vi "Point Tool Histogram Filter.vi"(4 "Range":cluster{"Lower value":sgl, "Upper value":sgl}={"Lower value"=162.0, "Upper value"=255.0}, 6 "Color threshold limits":T2, 8 "error in":errorcluster, 9 "Combo Box":string(combo), 10 "Subtraction Image":path, 11 "Image in":T1) -> (0 "error out":errorcluster, 3 "Image out":T1)   [LabVIEW 2020]
uses:
  <vilib>/vision/Image Controls.llb/IMAQ Image.ctl
  <vilib>/vision/NI_Vision_Development_Module.lvlib
panel:
  out "Image 2":T1(plugin-control)
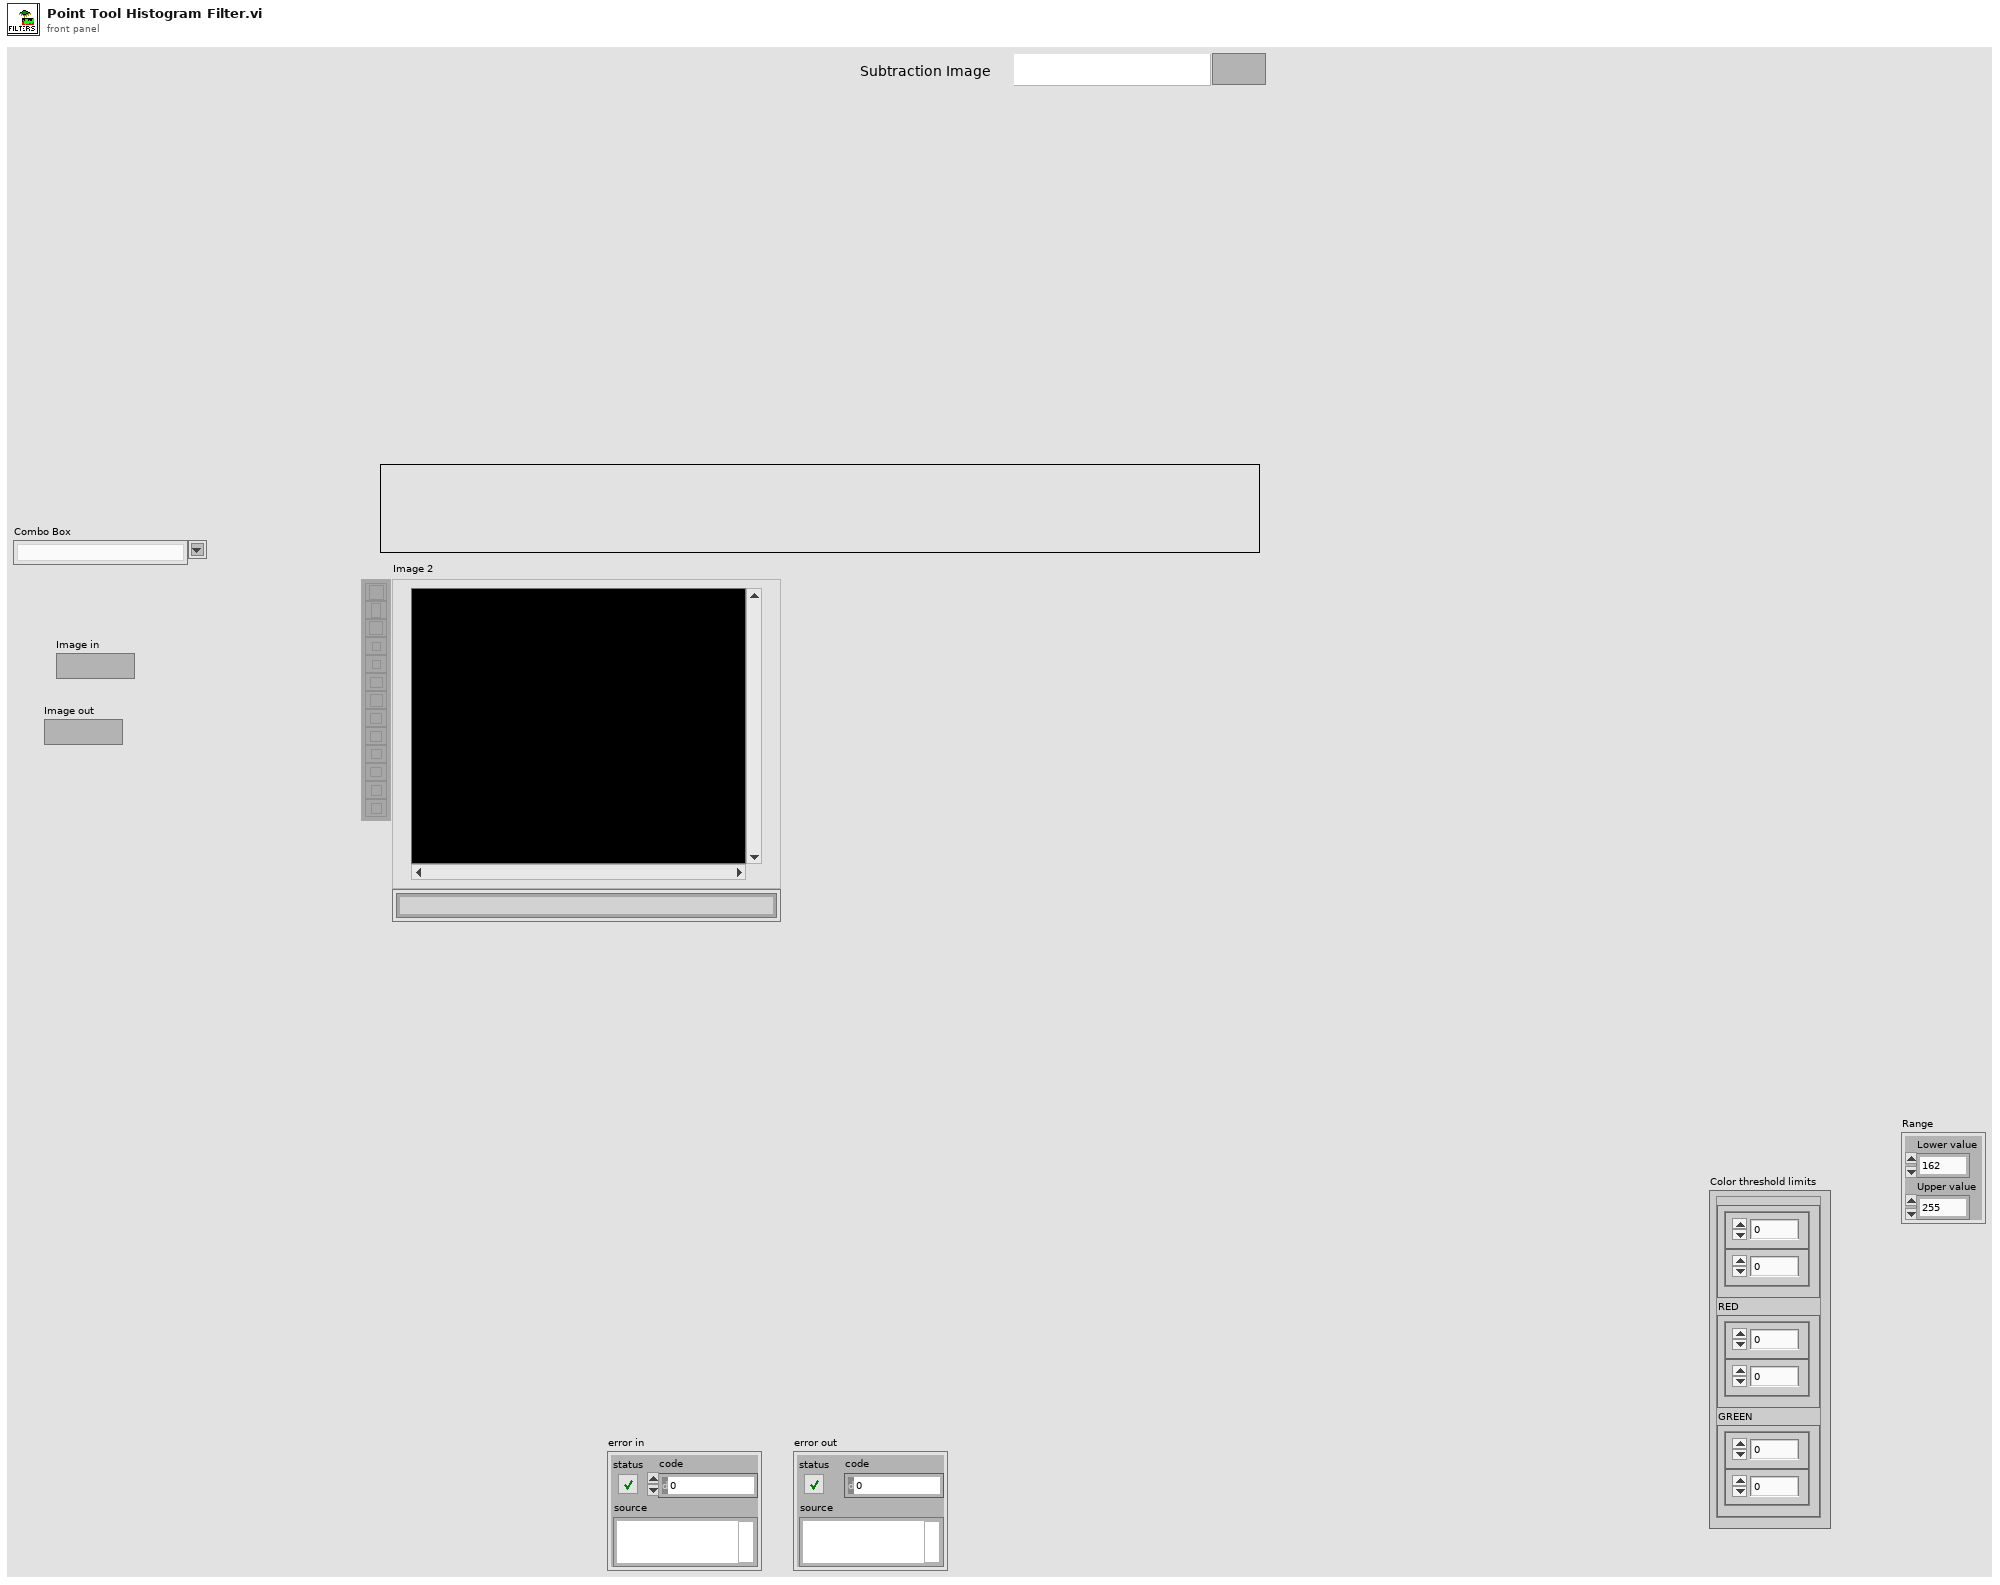
[diagram p1: front panel]
types:
  T1 = typedef "IMAQ Image.ctl" = refnum<image>
  T2 = cluster{"BLUE":cluster{"Numeric Control":dbl, "Numeric Control":dbl}, "RED":cluster{"Numeric Control":dbl, "Numeric Control":dbl}, "GREEN":cluster{"Numeric Control":dbl, "Numeric Control":dbl}}
  T3 = typedef "Image Type" = u32
  T4 = enum32{"Linear", "Log", "Exp", "Square", "Square root", "Power X", "Power 1/X"}
  T5 = cluster{"histogram":u32[], "Minimal Value":sgl, "Maximal Value":sgl, "Starting Value":sgl, "Interval Width":sgl, "Mean Value":sgl, "Standard  Variation":sgl, "Area (pixels)":i32}
  T6 = cluster{"Numeric Control":dbl, "Numeric Control":dbl}
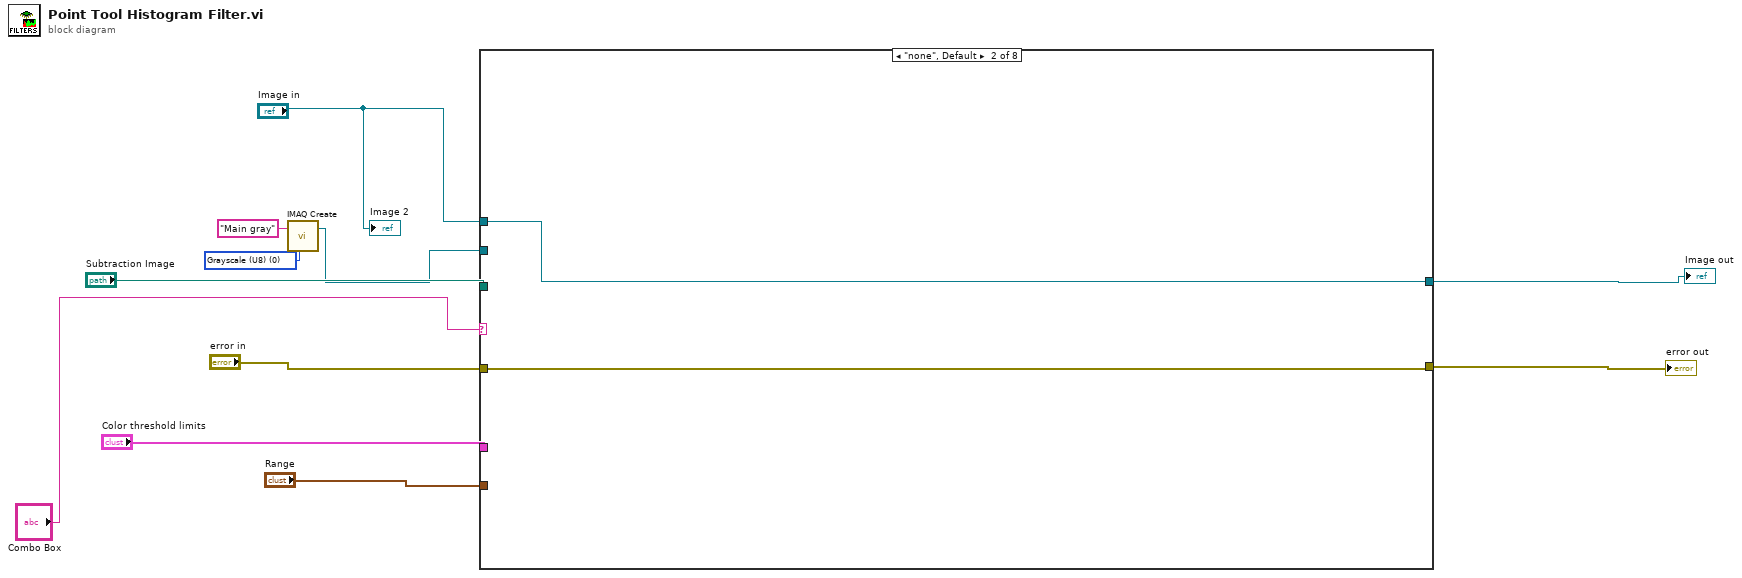
[diagram p0: block diagram]
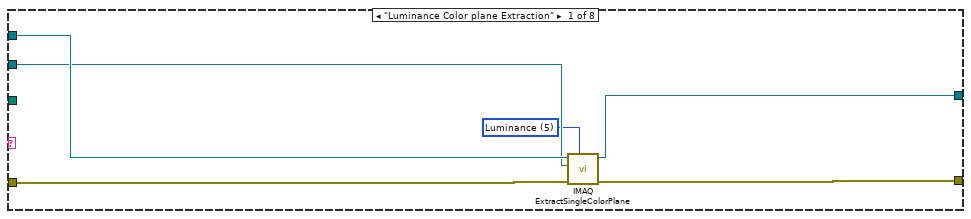
[diagram p2: hidden frame]
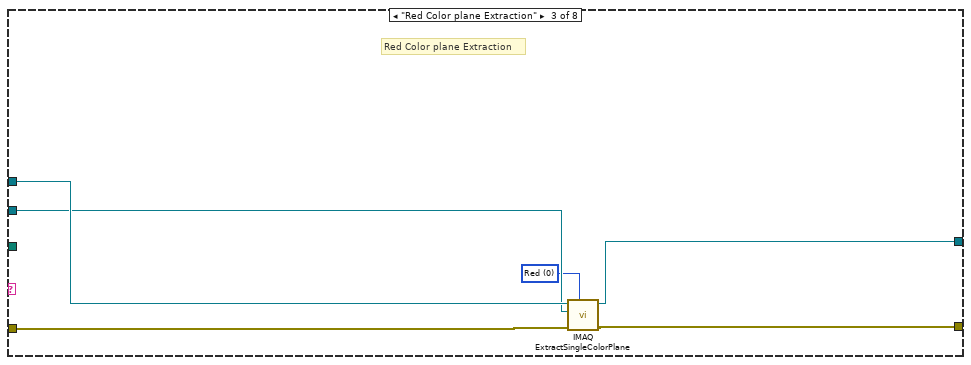
[diagram p3: hidden frame]
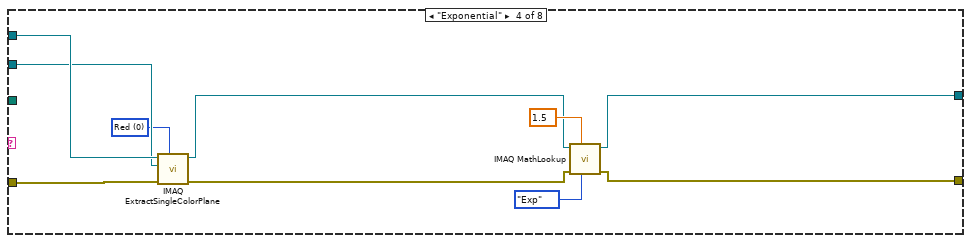
[diagram p4: hidden frame]
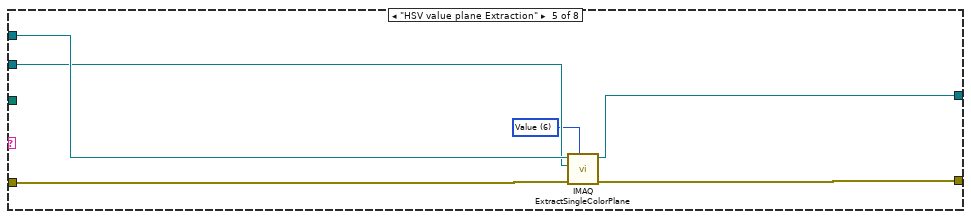
[diagram p5: hidden frame]
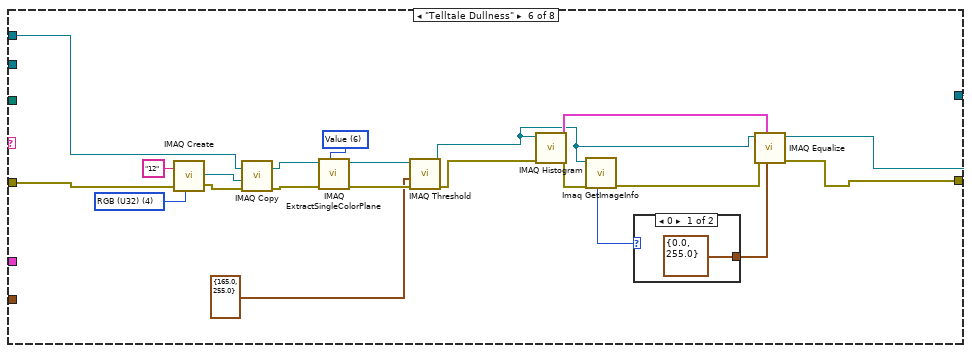
[diagram p6: hidden frame]
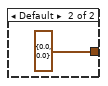
[diagram p7: hidden frame]
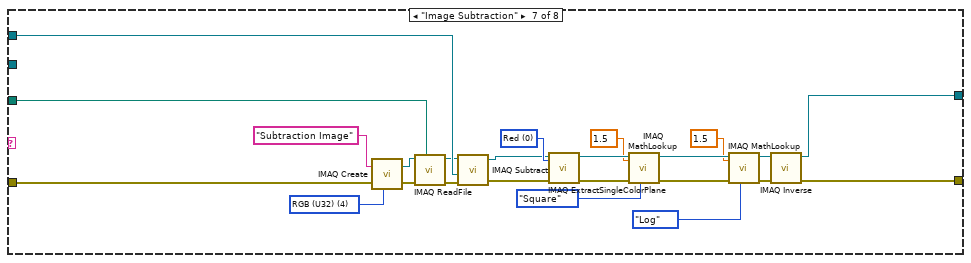
[diagram p8: hidden frame]
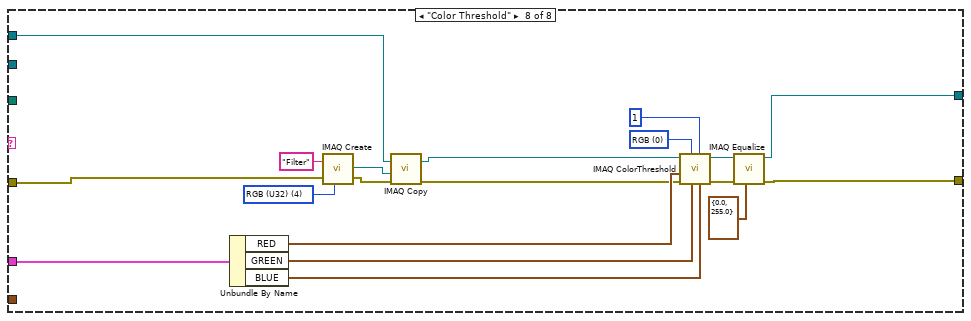
[diagram p9: hidden frame]
diagram:
  w5 = T3 0 items=["Grayscale (U8)", "Grayscale (I16)", "Grayscale (SGL)", "Complex (CSG)", "RGB (U32)", "HSL (U32)", "RGB (U64)", "Grayscale (U16)"] ("Image Type")
  n1 = call "IMAQ Create"("Image Name"="Main gray", "Image Type"=w5) -> ("New Image"=w4:T1)  [unwired: 3 in, 1 out]
  n2 = case shown="\"none\", Default" "Combo Box" {
    tunnel: [w16 w19 w20 w28 w40 w52 w88 w102] -> w11
    tunnel: "Image in" -> [w15 w18 w24 w34 w39 w44 w87 w90]
    tunnel: "Subtraction Image" -> [_ _ _ _ _ _ w86 _]
    tunnel: [w14 w18 w23 w26 w38 w51 w85 w97] -> w2
    tunnel: "error in" -> [w17 w19 w25 w35 w41 w46 w65 w95]
    tunnel: w4 -> [w13 _ w22 w33 w37 _ _ _]
    tunnel: "Color threshold limits" -> [_ _ _ _ _ _ _ w101]
    tunnel: "Range" -> [_ _ _ _ _ _ _ _]
    frame "Luminance Color plane Extraction" {
      w12 = 5 items=["Red", "Green", "Blue", "Hue", "Saturation", "Luminance", "Value", "Intensity"] ("Color Plane")
      n3 = call "IMAQ ExtractSingleColorPlane"("Color Plane"=w12, "error in (no error)"=w17, "Image Dst"=w13, "Image Src"=w15) -> ("error out"=w16:errorcluster, "Image Dst Out"=w14:T1)  [unwired: 6 in]
    }
    frame "none", Default {
    }
    frame "Red Color plane Extraction" {
      w21 = 0 items=["Red", "Green", "Blue", "Hue", "Saturation", "Luminance", "Value", "Intensity"] ("Color Plane")
      # "Red Color plane Extraction"
      n4 = call "IMAQ ExtractSingleColorPlane"("Color Plane"=w21, "error in (no error)"=w25, "Image Dst"=w22, "Image Src"=w24) -> ("error out"=w20:errorcluster, "Image Dst Out"=w23:T1)  [unwired: 6 in]
    }
    frame "Exponential" {
      w32 = 0 items=["Red", "Green", "Blue", "Hue", "Saturation", "Luminance", "Value", "Intensity"] ("Color Plane")
      n5 = call "IMAQ ExtractSingleColorPlane"("Color Plane"=w32, "error in (no error)"=w35, "Image Dst"=w33, "Image Src"=w34) -> ("error out"=w29:errorcluster, "Image Dst Out"=w27:T1)  [unwired: 6 in]
      n6 = call "IMAQ MathLookup"("Operator"=T4."Exp", "X Value"=sgl 1.5, "error in (no error)"=w29, "Image Src"=w27) -> ("error out"=w28:errorcluster, "Image Dst Out"=w26:T1)  [unwired: 3 in, 3 out]
    }
    frame "HSV value plane Extraction" {
      w36 = 6 items=["Red", "Green", "Blue", "Hue", "Saturation", "Luminance", "Value", "Intensity"] ("Color Plane")
      n7 = call "IMAQ ExtractSingleColorPlane"("Color Plane"=w36, "error in (no error)"=w41, "Image Dst"=w37, "Image Src"=w39) -> ("error out"=w40:errorcluster, "Image Dst Out"=w38:T1)  [unwired: 6 in]
    }
    frame "Telltale Dullness" {
      w48 = T3 4 items=["Grayscale (U8)", "Grayscale (I16)", "Grayscale (SGL)", "Complex (CSG)", "RGB (U32)", "HSL (U32)", "RGB (U64)", "Grayscale (U16)"] ("Image Type")
      w62 = 6 items=["Red", "Green", "Blue", "Hue", "Saturation", "Luminance", "Value", "Intensity"] ("Color Plane")
      n8 = call "IMAQ Create"("Image Name"="12", "Image Type"=w48, "error in (no error)"=w46) -> ("New Image"=w47:T1, "error out"=w50:errorcluster)  [unwired: 2 in]
      n9 = call "IMAQ Copy"("error in (no error)"=w50, "Image Dst"=w47, "Image Src"=w44) -> ("error out"=w45:errorcluster, "Image Dst Out"=w43:T1)  [unwired: 3 in]
      n10 = call "IMAQ ExtractSingleColorPlane"("Color Plane"=w62, "error in (no error)"=w45, "Image Src"=w43) -> ("error out"=w61:errorcluster, "Image Dst Out"=w60:T1)  [unwired: 1 in, 6 out]
      n11 = call "IMAQ Threshold"("error in (no error)"=w61, "Range"=cluster{"Lower value":sgl, "Upper value":sgl} {"Lower value"=165.0, "Upper value"=255.0}, "Image Src"=w60) -> ("error out"=w54:errorcluster, "Image Dst Out"=w53:T1)  [unwired: 3 in, 4 out]
      n12 = call "IMAQ Histogram"("error in (no error)"=w54, "Image"=w53) -> ("error out"=w57:errorcluster, "Histogram Report"=w59:T5)  [unwired: 3 in, 5 out]
      n13 = call "Imaq GetImageInfo"("error in (no error)"=w57, "Image"=w53) -> ("error out"=w56:errorcluster, "Image Type"=w58:T3)  [unwired: 8 out]
      n14 = case shown="0" w58 {
        tunnel: [cluster{"Minimum":sgl, "Maximum":sgl} {"Minimum"=0.0, "Maximum"=255.0} ("Range") cluster{"Minimum":sgl, "Maximum":sgl} {"Minimum"=0.0, "Maximum"=0.0} ("Range")] -> w55
        frame 0 {
        }
        frame Default {
        }
      }
      n15 = call "IMAQ Equalize"("Range"=w55, "Histogram Report"=w59, "error in (no error)"=w56, "Image Src"=w53) -> ("error out"=w52:errorcluster, "Image Dst Out"=w51:T1)  [unwired: 2 in, 4 out]
    }
    frame "Image Subtraction" {
      w72 = 0 items=["Red", "Green", "Blue", "Hue", "Saturation", "Luminance", "Value", "Intensity"] ("Color Plane")
      w81 = T3 4 items=["Grayscale (U8)", "Grayscale (I16)", "Grayscale (SGL)", "Complex (CSG)", "RGB (U32)", "HSL (U32)", "RGB (U64)", "Grayscale (U16)"] ("Image Type")
      n16 = call "IMAQ Create"("Image Name"="Subtraction Image", "Image Type"=w81, "error in (no error)"=w65) -> ("New Image"=w83:T1, "error out"=w84:errorcluster)  [unwired: 2 in]
      n17 = call "IMAQ ReadFile"("File Path"=w86, "error in (no error)"=w84, "Image"=w83) -> ("error out"=w80:errorcluster, "Image Out"=w79:T1)  [unwired: 4 in, 3 out]
      n18 = call "IMAQ Subtract"("Image Src A"=w79, "Image Src B"=w87, "error in (no error)"=w80) -> ("Image Dst Out"=w67:T1, "error out"=w66:errorcluster)  [unwired: 4 in]
      n19 = call "IMAQ ExtractSingleColorPlane"("Color Plane"=w72, "error in (no error)"=w66, "Image Src"=w67) -> ("error out"=w73:errorcluster, "Image Dst Out"=w74:T1)  [unwired: 1 in, 6 out]
      n20 = call "IMAQ MathLookup"("Operator"=T4."Square", "X Value"=sgl 1.5, "error in (no error)"=w73, "Image Src"=w74) -> ("error out"=w75:errorcluster, "Image Dst Out"=w76:T1)  [unwired: 3 in, 3 out]
      n21 = call "IMAQ MathLookup"("Operator"=T4."Log", "X Value"=sgl 1.5, "error in (no error)"=w75, "Image Src"=w76) -> ("error out"=w77:errorcluster, "Image Dst Out"=w78:T1)  [unwired: 3 in, 3 out]
      n22 = call "IMAQ Inverse"("error in (no error)"=w77, "Image Src"=w78) -> ("error out"=w88:errorcluster, "Image Dst Out"=w85:T1)  [unwired: 2 in, 6 out]
    }
    frame "Color Threshold" {
      w92 = T3 4 items=["Grayscale (U8)", "Grayscale (I16)", "Grayscale (SGL)", "Complex (CSG)", "RGB (U32)", "HSL (U32)", "RGB (U64)", "Grayscale (U16)"] ("Image Type")
      w107 = u16 0 items=["RGB", "HSL", "HSV", "HSI"] ("Color Mode (Color Threshold 1)")
      n23 = Unbundle By Name(w101) -> ("RED"=w100:T6, "GREEN"=w99:T6, "BLUE"=w98:T6)
      n24 = call "IMAQ Create"("Image Name"="Filter", "Image Type"=w92, "error in (no error)"=w95) -> ("New Image"=w91:T1, "error out"=w96:errorcluster)  [unwired: 2 in]
      n25 = call "IMAQ Copy"("error in (no error)"=w96, "Image Dst"=w91, "Image Src"=w90) -> ("error out"=w94:errorcluster, "Image Dst Out"=w89:T1)  [unwired: 3 in]
      n26 = call "IMAQ ColorThreshold"("Blue or Luma or Val or Inten Range"=w98, "Replace Value"=1, "Green or Sat Range"=w99, "Color Mode"=w107, "error in (no error)"=w94, "Red or Hue Range"=w100, "Image Src"=w89) -> ("error out"=w103:errorcluster, "Image Dst Out"=w104:T1)  [unwired: 1 in, 2 out]
      n27 = call "IMAQ Equalize"("Range"=cluster{"Minimum":sgl, "Maximum":sgl} {"Minimum"=0.0, "Maximum"=255.0}, "error in (no error)"=w103, "Image Src"=w104) -> ("error out"=w102:errorcluster, "Image Dst Out"=w97:T1)  [unwired: 3 in, 4 out]
    }
  }
  "error out" <- w11
  "Image out" <- w2
  "Image 2" <- "Image in"
